vi "Subscribe_QMH.vi"() -> ()   [LabVIEW 2015]
uses:
  Program Files/National Instruments/LabVIEW 2015/ProjectTemplates/Source/Core/Queued Message Handler/support/Message Queue/Subscribe_Data.ctl
  <vilib>/daq.io/MQTT LabVIEW Client/Controls/QoS.ctl
  <vilib>/daq.io/MQTT LabVIEW Client/Controls/Connect_Flags.ctl
  <vilib>/daq.io/MQTT LabVIEW Client/Controls/DUP_Flag.ctl
  <vilib>/daq.io/MQTT LabVIEW Client/Controls/Retain_Flag.ctl
  <vilib>/daq.io/MQTT LabVIEW Client/Controls/Connection_Return_Codes.ctl
  Data_Save.ctl
  Program Files/National Instruments/LabVIEW 2015/ProjectTemplates/Source/Core/Queued Message Handler/support/Message Queue/Enqueue Message (Single).vi
  <vilib>/Utility/error.llb/Error Cluster From Error Code.vi
  <vilib>/ErrorRing/Error Ring.xnode
  Program Files/National Instruments/LabVIEW 2015/ProjectTemplates/Source/Core/Queued Message Handler/support/User Event - Stop/User Event - Stop.lvlib
  Program Files/National Instruments/LabVIEW 2015/ProjectTemplates/Source/Core/Queued Message Handler/support/Message Queue/Message Queue.lvlib
  <vilib>/daq.io/MQTT LabVIEW Client/MQTT_Functions.lvlib
panel:
  in  "append to file? (new file:F)":bool=TRUE
  out "Published Data":string[][](array[string])
  out "Samples Collected":i32
  in  "Sample Period(s)":dbl=1.0
  out "Connection Status":T1=enum."Connection refused: not authorized"
  out "Main Display":string
  in  "?":T2={"Subscriber ID"="GETmyRIO", "MQTT Broker"={"address (IP)"="52.37.169.179", "port"=1883}, "Subscription Info Array"=[{"Topic"="a/b", "QoS"=enum."At least once"}], "Connect Flags"={"user name"=FALSE, "password"=FALSE, "will retain"=FALSE, "will flag"=FALSE, "clean session"=TRUE, "reserved"=FALSE, "will QoS"=enum."At most once"}, "Connect Meta"={"QoS"=enum."At most once", "DUP"=FALSE, "Retain"=FALSE, "Keep Alive (sec)"=60}, "Exit"=refnum, "connection ID out"=refnum, "Main Display"=""}
  in  "Exit":bool
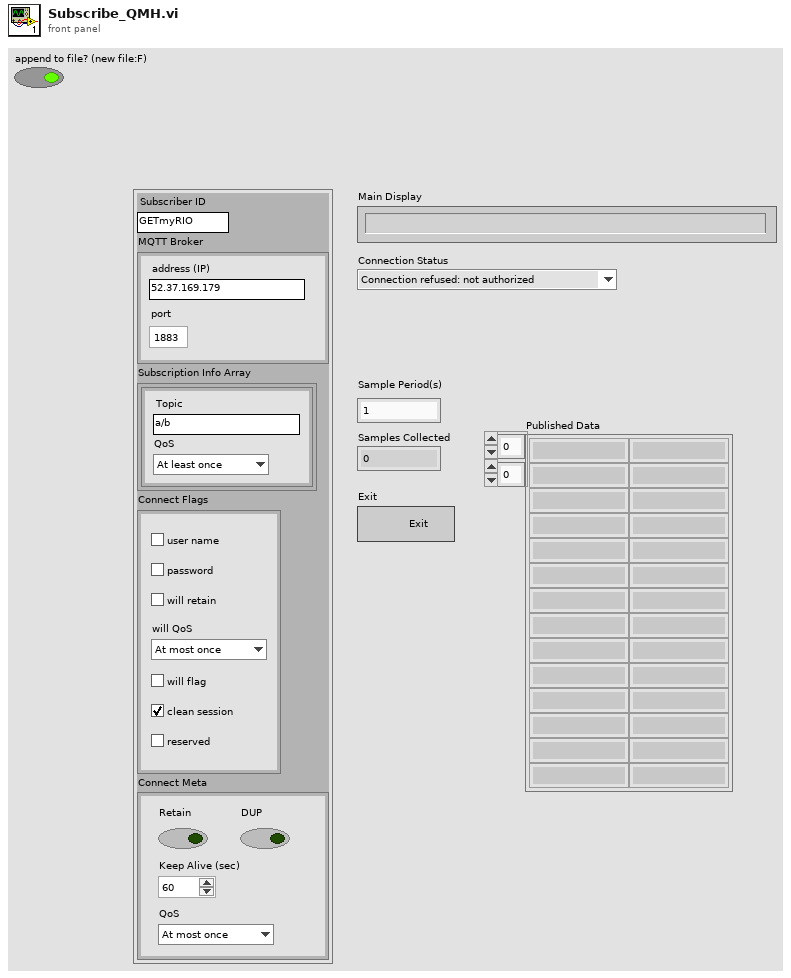
[diagram p1: front panel]
types:
  T1 = typedef "MQTT_Functions.lvlib/Connection_Return_Codes.ctl" = enum16{"Connection accepted", "Connection refused: unacceptable protocol version", "Connection refused: identifier rejected", "Connection refused: Server unavailable", "Connection refused: bad user name or password", "Connection refused: not authorized"}
  T2 = typedef "Subscribe_Data.ctl" = cluster{"Subscriber ID":string, "MQTT Broker":cluster{"address (IP)":string, "port":u16}, "Subscription Info Array":cluster{"Topic":string, "QoS":T3}[], "Connect Flags":T4, "Connect Meta":cluster{"QoS":T3, "DUP":T5, "Retain":T6, "Keep Alive (sec)":u16}, "Exit":refnum<vi>, "connection ID out":refnum<k5>, "Main Display":string}
  T3 = typedef "MQTT_Functions.lvlib/QoS.ctl" = enum8{"At most once", "At least once", "Exactly once", "Reserved"}
  T4 = typedef "MQTT_Functions.lvlib/Connect_Flags.ctl" = cluster{"user name":bool, "password":bool, "will retain":bool, "will flag":bool, "clean session":bool, "reserved":bool, "will QoS":T3}
  T5 = typedef "MQTT_Functions.lvlib/DUP_Flag.ctl" = bool
  T6 = typedef "MQTT_Functions.lvlib/Retain_Flag.ctl" = bool
  T7 = typedef "Data_Save.ctl" = cluster{"Data Columns":string, "Raw Data":string, "file path (dialog if empty)":path, "Append File":refnum<vi>}
  T8 = typedef "Queues.ctl" = cluster{"Suscribe":refnum<queue>, "Display/Save Data":refnum<queue>}
  T9 = cluster{"QoS":T3, "DUP":T5, "Retain":T6, "Keep Alive (sec)":u16}
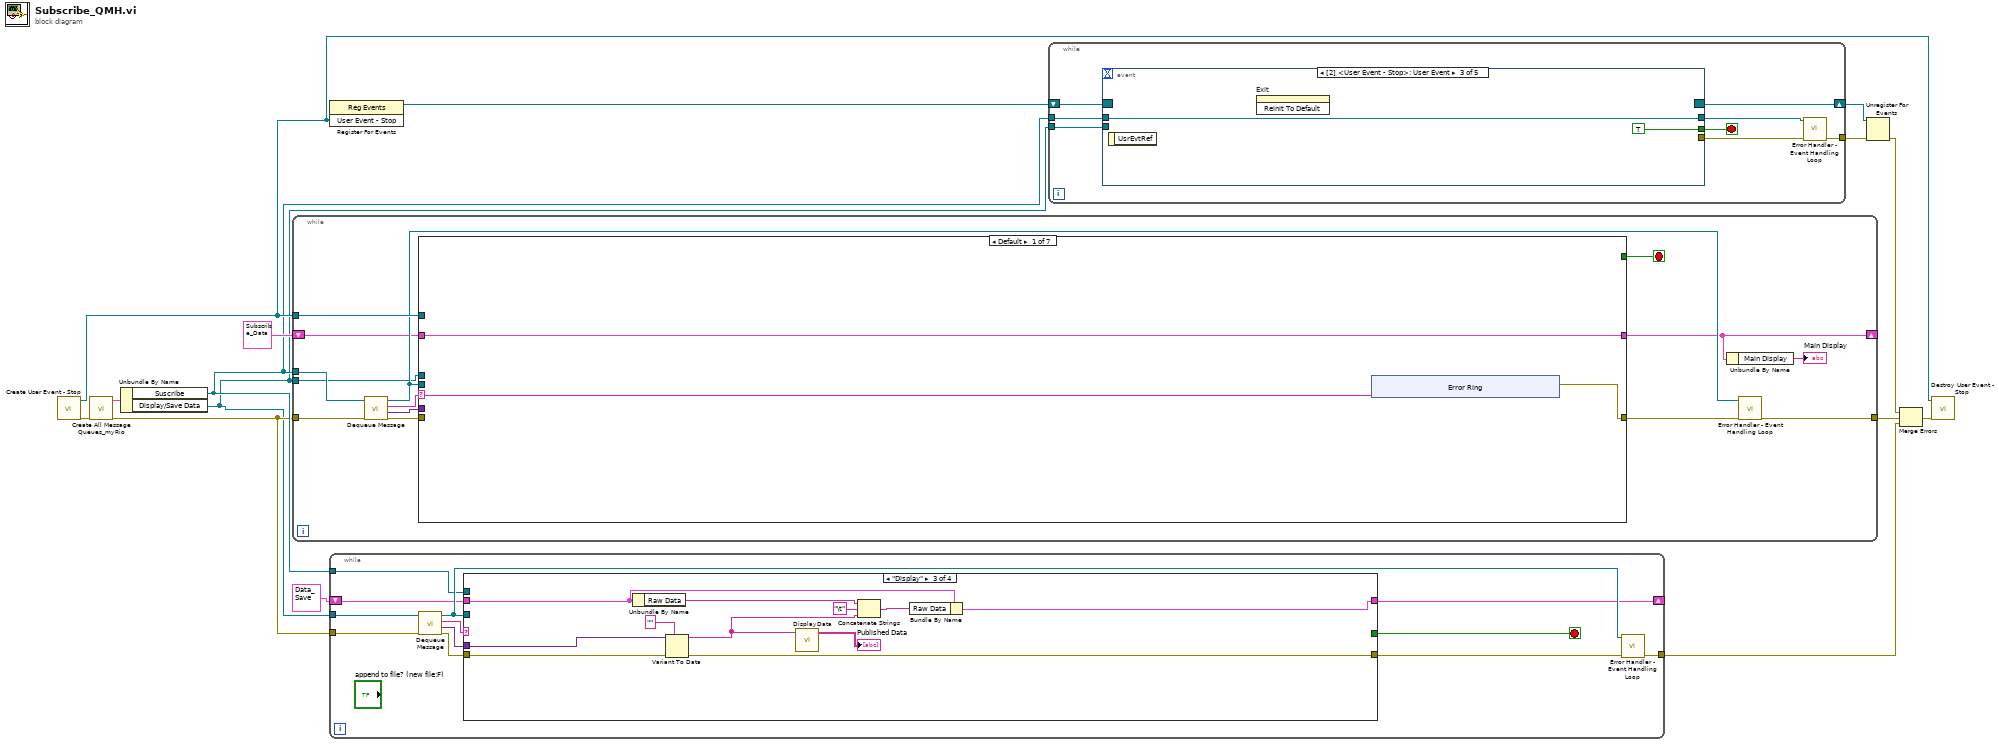
[diagram p0: block diagram]
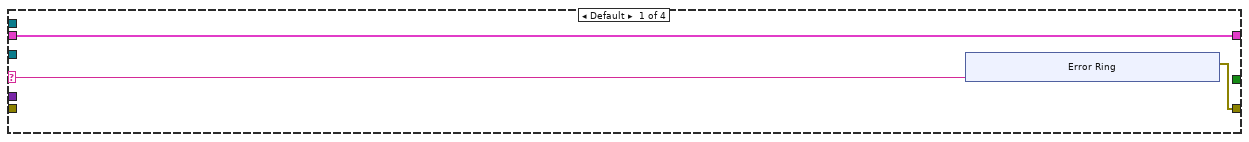
[diagram p2: hidden frame]
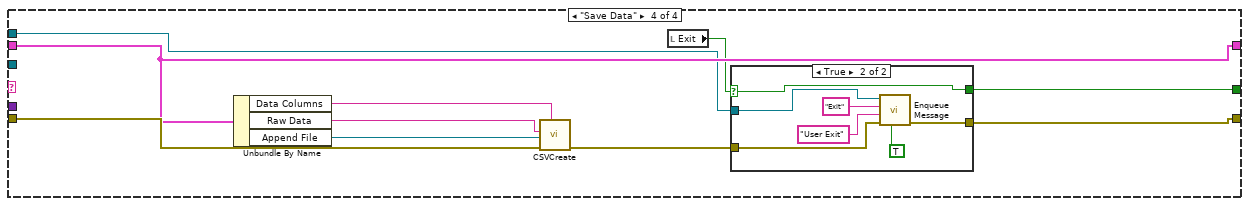
[diagram p4: hidden frame]
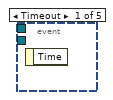
[diagram p6: hidden frame]
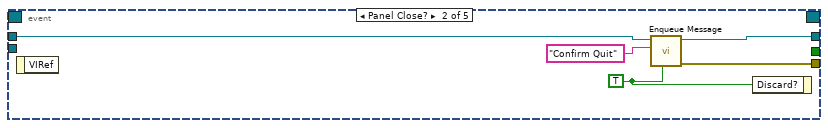
[diagram p7: hidden frame]
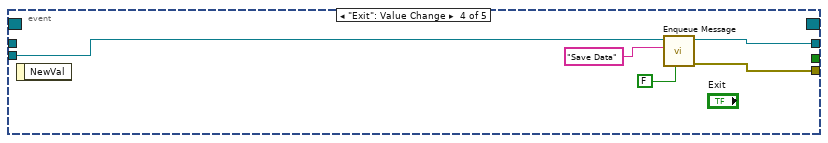
[diagram p8: hidden frame]
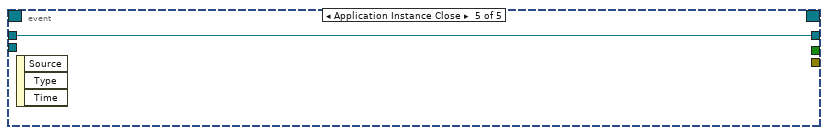
[diagram p9: hidden frame]
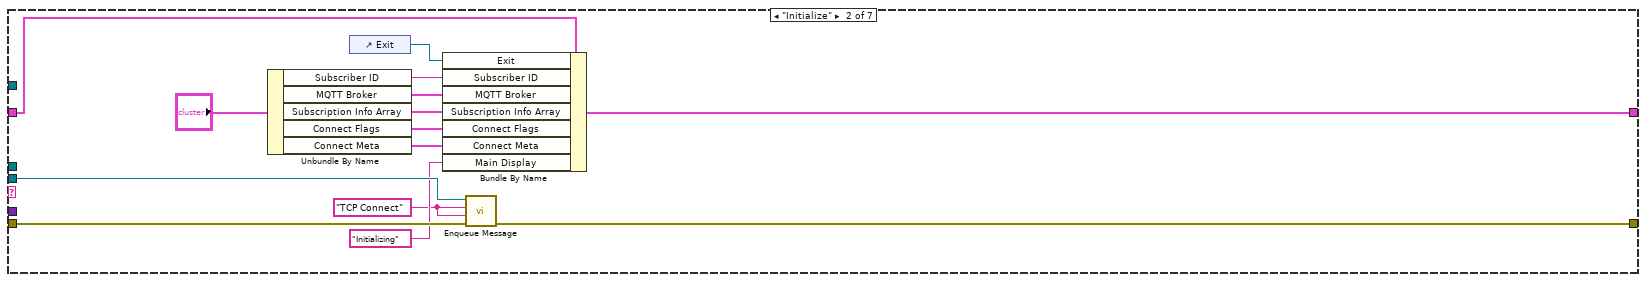
[diagram p10: hidden frame]
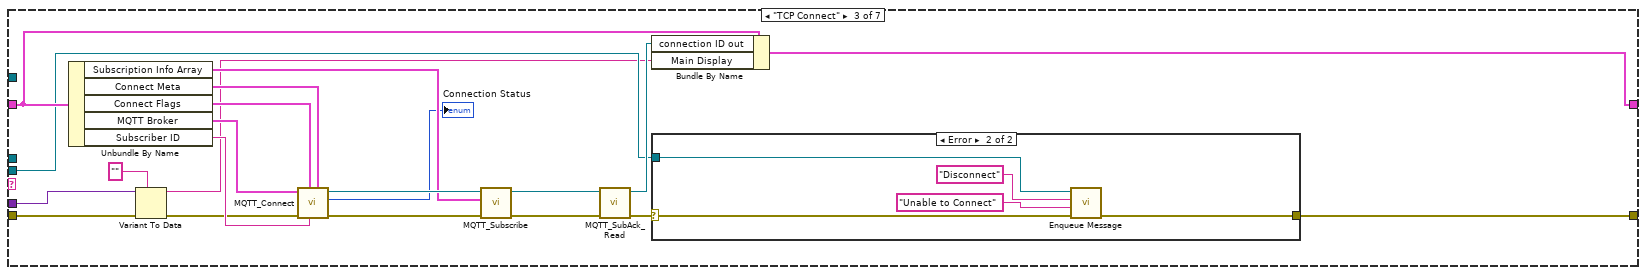
[diagram p11: hidden frame]
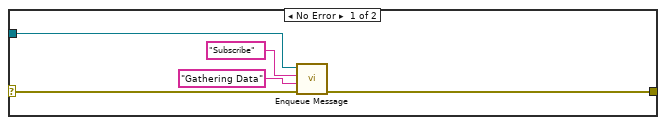
[diagram p12: hidden frame]
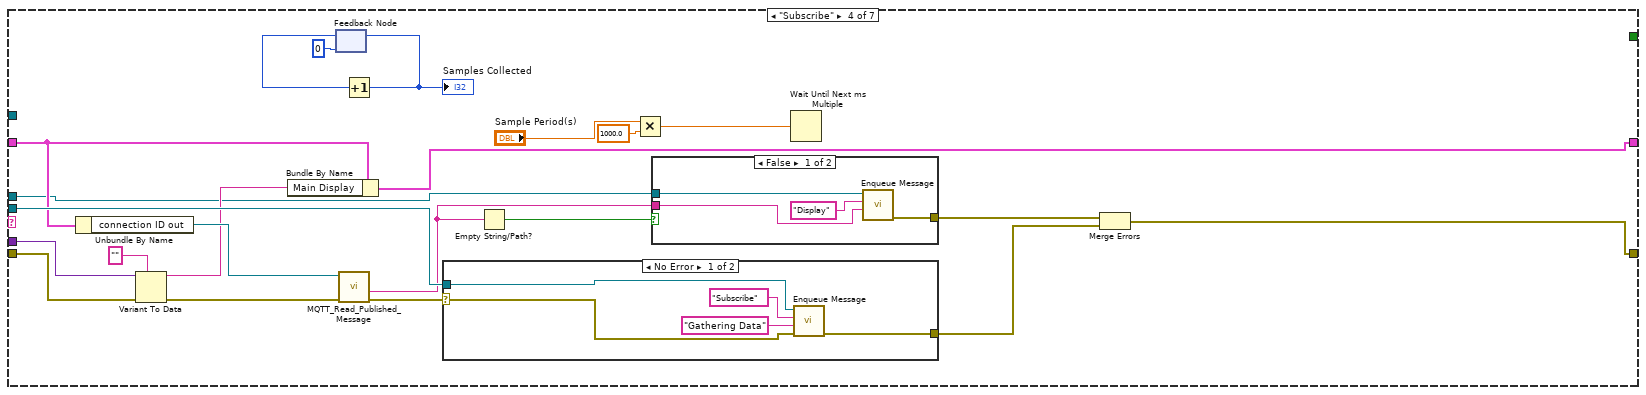
[diagram p13: hidden frame]
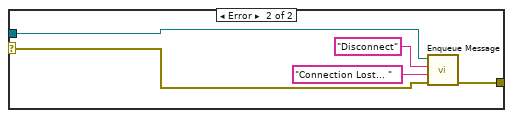
[diagram p14: hidden frame]
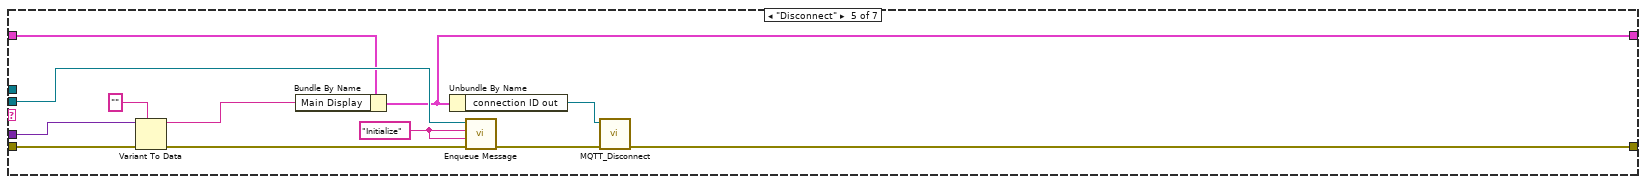
[diagram p16: hidden frame]
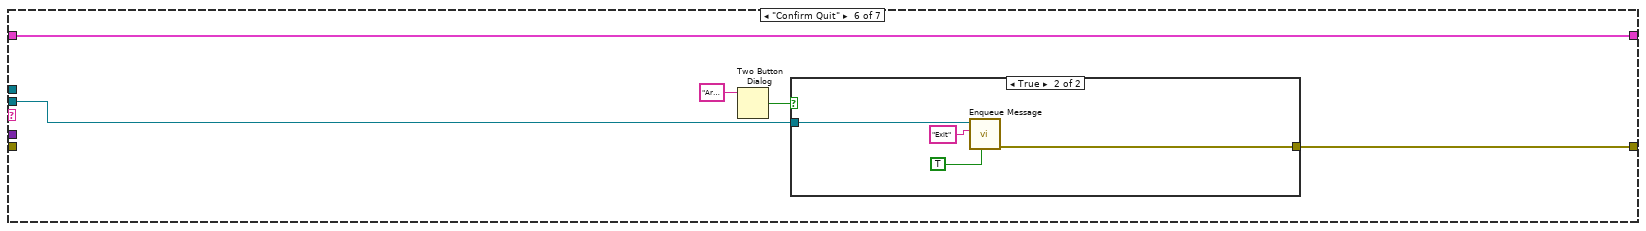
[diagram p17: hidden frame]
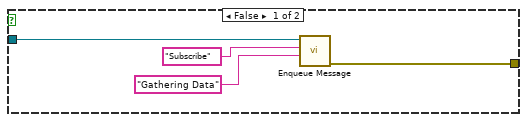
[diagram p18: hidden frame]
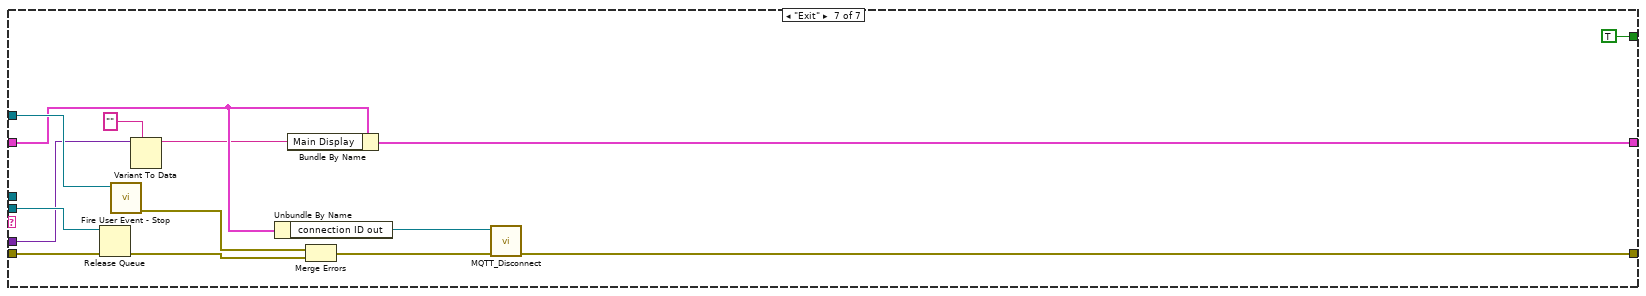
[diagram p19: hidden frame]
diagram:
  n1 = call "Create User Event - Stop.vi"() -> ("error out"=w15:errorcluster, "User Event - Stop"=w6:refnum<user-event>)  [unwired: 10 in]
  n2 = call "Create All Message Queues_myRio.vi"("error in (no error)"=w15) -> ("error out"=w4:errorcluster, "Queues"=w7:T8)  [unwired: 9 in]
  n3 = Unbundle By Name(w7) -> ("Suscribe"=w5:refnum<queue>, "Display/Save Data"=w1:refnum<queue>)
  n4 = while {
    tunnel: w4 -> [w29]
    tunnel: [w28] -> w9
    tunnel: w6 -> [w25]
    shift-right: [w18] -> _
    shift-left: T2 {"Subscriber ID"="GETmyRIO", "MQTT Broker"={"address (IP)"="52.37.169.179", "port"=1883}, "Subscription Info Array"=[{"Topic"="a/b", "QoS"=enum."At least once"}], "Connect Flags"={"user name"=FALSE, "password"=FALSE, "will retain"=FALSE, "will flag"=FALSE, "clean session"=TRUE, "reserved"=FALSE, "will QoS"=enum."At most once"}, "Connect Meta"={"QoS"=enum."At most once", "DUP"=FALSE, "Retain"=FALSE, "Keep Alive (sec)"=60}, "Exit"=refnum, "connection ID out"=refnum, "Main Display"=""} -> [w20]
    tunnel: w5 -> [w19]
    tunnel: w1 -> [w16]
    stop <- w22 stop-if-true
    n5 = call "Dequeue Message.vi"("error in (no error)"=w29, "Message Queue"=w19) -> ("error out"=w23:errorcluster, "Message Data"=w27:variant, "Message"=w26:string, "dup Message Queue"=w24:refnum<queue>)  [unwired: 6 in]
    n6 = case shown="Default" w26 {
      selector: w26 -> [w32 _ _ _ _ _ _]
      tunnel: w27 -> [_ _ w58 w92 w127 _ w150]
      tunnel: w25 -> [_ _ _ _ _ _ w159]
      tunnel: w24 -> [_ w44 w60 w101 w130 w137 w158]
      tunnel: w23 -> [_ w43 w57 w97 w125 _ w157]
      tunnel: [_ _ _ _ _ _ TRUE] -> w22
      tunnel: [w31 w42 w59 w99 w131 w136 w152] -> w21
      tunnel: w20 -> [w30 w52 w63 w94 w122 w133 w148]
      tunnel: [w30 w51 w62 w93 w121 w133 w147] -> w18
      tunnel: w16 -> [_ _ _ w87 _ _ _]
      frame Default {
        n7 = xnode "Error Ring"("parameter 0"=w32) -> ("error out"=w31:errorcluster)
      }
      frame "Initialize" {
        w40 = "TCP Connect" ("Message")
        n8 = Unbundle By Name("?") -> ("Subscriber ID"=w49:string, "MQTT Broker"=w48:cluster{"address (IP)":string, "port":u16}, "Subscription Info Array"=w47:cluster{"Topic":string, "QoS":T3}[], "Connect Flags"=w46:T4, "Connect Meta"=w45:T9)
        n9 = control-ref of="Exit"() -> (w53:refnum<vi>)
        n10 = Bundle By Name(cluster=w52, "Exit"=w53, "Subscriber ID"=w49, "MQTT Broker"=w48, "Subscription Info Array"=w47, "Connect Flags"=w46, "Connect Meta"=w45, "Main Display"="Initializing" ("Message")) -> (w51:T2)
        n11 = call-poly "Enqueue Message.vi"("error in (no error)"=w43, "Message Data"=w40, "Message"=w40, "Message Queue"=w44) -> ("error out"=w42:errorcluster)  [unwired: 6 in, 1 out]
      }
      frame "TCP Connect" {
        n12 = Unbundle By Name(w63) -> ("Subscription Info Array"=w66:cluster{"Topic":string, "QoS":T3}[], "Connect Meta"=w67:T9, "Connect Flags"=w68:T4, "MQTT Broker"=w69:cluster{"address (IP)":string, "port":u16}, "Subscriber ID"=w70:string)
        n13 = Variant To Data(error in=w57, type="", Variant=w58) -> (data=w55:string, error out=w54:errorcluster)
        n14 = call <vilib>:"MQTT_Connect.vi"("Connect Meta"=w67, "Client ID"=w70, "Connect Flags"=w68, "error in (no error)"=w54, "MQTT Broker"=w69) -> ("error out"=w72:errorcluster, "Connection Status"=→"Connection Status":T1, "connection ID out"=w71:refnum<k5>)  [unwired: 4 in]
        n15 = call <vilib>:"MQTT_Subscribe.vi"("error in (no error)"=w72, "Subscription Info Array"=w66, "connection ID"=w71) -> ("error out"=w74:errorcluster, "connection ID out"=w73:refnum<k5>)  [unwired: 7 in]
        n16 = call <vilib>:"MQTT_SubAck_Read.vi"("error in (no error)"=w74, "connection ID"=w73) -> ("error out"=w61:errorcluster, "connection ID out"=w64:refnum<k5>)  [unwired: 7 in, 1 out]
        n17 = Bundle By Name(cluster=w63, "connection ID out"=w64, "Main Display"=w55) -> (w62:T2)
        n18 = case shown="Error" w61 {
          selector: w61 -> [w77 w83]
          tunnel: w60 -> [w78 w84]
          tunnel: [w76 w82] -> w59
          frame No Error {
            n19 = call-poly "Enqueue Message.vi"("error in (no error)"=w77, "Message Data"="Gathering Data" ("Message"), "Message"="Subscribe", "Message Queue"=w78) -> ("error out"=w76:errorcluster)  [unwired: 6 in, 1 out]
          }
          frame Error {
            n20 = call-poly "Enqueue Message.vi"("error in (no error)"=w83, "Message Data"="Unable to Connect" ("Message"), "Message"="Disconnect", "Message Queue"=w84) -> ("error out"=w82:errorcluster)  [unwired: 6 in, 1 out]
          }
        }
      }
      frame "Subscribe" {
        n21 = Unbundle By Name(w94) -> ("connection ID out"=w102:refnum<k5>)
        n22 = Variant To Data(error in=w97, type="", Variant=w92) -> (data=w95:string, error out=w96:errorcluster)
        n23 = Bundle By Name(cluster=w94, "Main Display"=w95) -> (w93:T2)
        n24 = feedback #1(0) -> (w104:i32)
        n25 = call <vilib>:"MQTT_Read_Published_Message.vi"("error in (no error)"=w96, "connection ID"=w102) -> ("error out"=w85:errorcluster, "Message"=w88:string)  [unwired: 4 in, 4 out]
        n26 = Increment(x=w104) -> (x+1=w105:i32)
        "Samples Collected" <- w105
        n27 = feedback-in #1(w105) -> ()
        n28 = case shown="No Error" w85 {
          selector: w85 -> [w108 w113]
          tunnel: w101 -> [w111 w116]
          tunnel: [w109 w115] -> w100
          frame No Error {
            n29 = call-poly "Enqueue Message.vi"("error in (no error)"=w108, "Message Data"="Gathering Data" ("Message"), "Message"="Subscribe", "Message Queue"=w111) -> ("error out"=w109:errorcluster)  [unwired: 6 in, 1 out]
          }
          frame Error {
            n30 = call-poly "Enqueue Message.vi"("error in (no error)"=w113, "Message Data"="Connection Lost... " ("Message"), "Message"="Disconnect", "Message Queue"=w116) -> ("error out"=w115:errorcluster)  [unwired: 6 in, 1 out]
          }
        }
        n31 = Empty String/Path?(string/path=w88) -> (empty?=w103:bool)
        n32 = Multiply(x="Sample Period(s)", y=1000.0 ("milliseconds to wait")) -> (x*y=w89:dbl)
        n33 = case shown="False" w103 {
          tunnel: w88 -> [w118 _]
          tunnel: w87 -> [w120 _]
          tunnel: [w117 _] -> w86
          frame False {
            n34 = call-poly "Enqueue Message.vi"("Message Data"=w118, "Message"="Display", "Message Queue"=w120) -> ("error out"=w117:errorcluster)  [unwired: 7 in, 1 out]
          }
          frame True {
          }
        }
        n35 = Wait Until Next ms Multiple(millisecond multiple=w89) -> ()  [unwired: 1 out]
        n36 = Merge Errors(w86, w100) -> (w99:errorcluster)
      }
      frame "Disconnect" {
        w128 = "Initialize" ("Message")
        n37 = Variant To Data(error in=w125, type="", Variant=w127) -> (data=w123:string, error out=w124:errorcluster)
        n38 = Bundle By Name(cluster=w122, "Main Display"=w123) -> (w121:T2)
        n39 = Unbundle By Name(w121) -> ("connection ID out"=w132:refnum<k5>)
        n40 = call-poly "Enqueue Message.vi"("error in (no error)"=w124, "Message Data"=w128, "Message"=w128, "Message Queue"=w130) -> ("error out"=w129:errorcluster)  [unwired: 6 in, 1 out]
        n41 = call <vilib>:"MQTT_Disconnect.vi"("error in (no error)"=w129, "connection ID"=w132) -> ("error out"=w131:errorcluster)  [unwired: 9 in]
      }
      frame "Confirm Quit" {
        n42 = Two Button Dialog(message="Are you sure you want to quit?") -> (T button?=w134:bool)  [unwired: 2 in]
        n43 = case shown="True" w134 {
          tunnel: w137 -> [w141 w145]
          tunnel: [w139 w143] -> w136
          frame False {
            n44 = call-poly "Enqueue Message.vi"("Message Data"="Gathering Data" ("Message"), "Message"="Subscribe", "Message Queue"=w141) -> ("error out"=w139:errorcluster)  [unwired: 7 in, 1 out]
          }
          frame True {
            n45 = call-poly "Enqueue Message.vi"("Priority Message? (F)"=TRUE, "Message"="Exit", "Message Queue"=w145) -> ("error out"=w143:errorcluster)  [unwired: 7 in, 1 out]
          }
        }
      }
      frame "Exit" {
        n46 = Release Queue(queue=w158, error in (no error)=w157) -> (error out=w155:errorcluster)  [unwired: 1 in, 2 out]
        n47 = call "Fire User Event - Stop.vi"("User Event - Stop"=w159) -> ("error out"=w156:errorcluster)  [unwired: 10 in]
        n48 = Variant To Data(type="", Variant=w150) -> (data=w146:string)  [unwired: 1 in, 1 out]
        n49 = Unbundle By Name(w148) -> ("connection ID out"=w151:refnum<k5>)
        n50 = Bundle By Name(cluster=w148, "Main Display"=w146) -> (w147:T2)
        n51 = Merge Errors(w156, w155) -> (w153:errorcluster)
        n52 = call <vilib>:"MQTT_Disconnect.vi"("error in (no error)"=w153, "connection ID"=w151) -> ("error out"=w152:errorcluster)  [unwired: 9 in]
      }
    }
    n53 = Unbundle By Name(w18) -> ("Main Display"=→"Main Display":string)
    n54 = call "Error Handler - Event Handling Loop.vi"("error in (no error)"=w21, "Message Queue"=w24) -> ("dup error in"=w28:errorcluster)  [unwired: 8 in, 1 out]
  }
  n55 = register-events(w6) -> (reference out=w14:refnum<event-registration>)  [unwired: 2 in, 1 out]
  n56 = while {
    tunnel: w1 -> [w171]
    tunnel: w5 -> [w160]
    tunnel: w4 -> [w170]
    tunnel: [w165] -> w3
    shift-right: [w162] -> _
    shift-left: T7 {"Data Columns"="Timestamp,Wind Direction,Wind Speed,Air Temperature,Internal Temperature,Relative Humidity,Air Pressure,Rain Accumulation, Rain Duration, Rain Intensity,Hail Duration, Hail Intensity, Supply Voltage, Solar Irradiance", "Raw Data"="", "file path (dialog if empty)"=path "C:/Users/jas921/Desktop/Labview Test Data/test.csv", "Append File"=refnum} ("Display/Save Data") -> [w163]
    stop <- w161 stop-if-true
    n57 = call "Dequeue Message.vi"("error in (no error)"=w170, "Message Queue"=w171) -> ("error out"=w169:errorcluster, "Message Data"=w168:variant, "Message"=w167:string, "dup Message Queue"=w164:refnum<queue>)  [unwired: 6 in]
    n58 = case shown="\"Display\"" w167 {
      selector: w167 -> [w174 _ _ _]
      tunnel: w169 -> [_ w183 w192 w204]
      tunnel: w168 -> [_ _ w193 _]
      tunnel: w164 -> [_ _ _ _]
      tunnel: [w173 w183 w184 w197] -> w166
      tunnel: w163 -> [w172 w182 w186 w203]
      tunnel: [w172 w182 w188 w203] -> w162
      tunnel: [_ _ _ w199] -> w161
      tunnel: w160 -> [_ _ _ w198]
      frame Default {
        n59 = xnode "Error Ring"("parameter 0"=w174) -> ("error out"=w173:errorcluster)
      }
      frame "Wait" {
      }
      frame "Display" {
        n60 = Unbundle By Name(w186) -> ("Raw Data"=w185:string)
        n61 = Variant To Data(error in=w192, type="", Variant=w193) -> (data=w189:string, error out=w184:errorcluster)
        n62 = call "DisplayData.vi"("CSV Input"=w189) -> ("Published Data"=→"Published Data":string[][])  [unwired: 10 in]
        n63 = Concatenate Strings(w185, "\t", w189) -> (w187:string)
        n64 = Bundle By Name(cluster=w186, "Raw Data"=w187) -> (w188:T7)
      }
      frame "Save Data" {
        n65 = Unbundle By Name(w203) -> ("Data Columns"=w202:string, "Raw Data"=w201:string, "Append File"=w195:refnum<vi>)
        n66 = call "CSVCreate.vi"("Header"=w202, "error in"=w204, "Append File"=w195, "Data Input"=w201) -> ("error out"=w196:errorcluster)  [unwired: 6 in, 1 out]
        n67 = local read "Exit"() -> (w200:bool)
        n68 = case shown="True" w200 {
          selector: w200 -> [_ w212]
          tunnel: [_ w212] -> w199
          tunnel: w198 -> [_ w211]
          tunnel: [w205 w208] -> w197
          tunnel: w196 -> [w205 w207]
          frame False {
          }
          frame True {
            n69 = call-poly "Enqueue Message.vi"("Priority Message? (F)"=TRUE, "error in (no error)"=w207, "Message Data"="User Exit" ("Message"), "Message"="Exit", "Message Queue"=w211) -> ("error out"=w208:errorcluster)  [unwired: 5 in, 1 out]
          }
        }
      }
    }
    n70 = call "Error Handler - Event Handling Loop.vi"("error in (no error)"=w166, "Message Queue"=w164) -> ("dup error in"=w165:errorcluster)  [unwired: 8 in, 1 out]
  }
  n71 = while {
    tunnel: w5 -> [w220]
    tunnel: [w217] -> w12
    shift-right: [w215] -> w13
    shift-left: w14 -> [w216]
    tunnel: w1 -> [w213]
    stop <- w214 stop-if-true
    n72 = event shown="[2] <User Event - Stop>: User Event" {
      selector: w216 -> [_ _ _ _ _]
      dyn-events: [_ _ _ _ _] -> w215
      timeout: _ -> [_ _ _ _ _]
      tunnel: w220 -> [_ w224 w226 _ w233]
      tunnel: [_ w223 w226 w232 w233] -> w219
      tunnel: [_ w222 _ w229 _] -> w218
      tunnel: [_ _ TRUE _ _] -> w214
      tunnel: w213 -> [_ _ _ w228 _]
      event Timeout {
        n73 = event-data() -> ()  [unwired: 1 in, 1 out]
      }
      event Panel Close? {
        w221 = TRUE
        n74 = event-data() -> ()  [unwired: 1 in, 1 out]
        n75 = call-poly "Enqueue Message.vi"("Priority Message? (F)"=w221, "Message"="Confirm Quit", "Message Queue"=w224) -> ("error out"=w222:errorcluster, "dup Message Queue"=w223:refnum<queue>)  [unwired: 7 in]
        n76 = event-data("Discard?"=w221) -> ()  [unwired: 1 in, 1 out]
      }
      event User Event {
        n77 = event-data() -> ()  [unwired: 1 in, 1 out]
        n78 = invoke on="Exit" class="Bool (strict)" method="Reinit To Default"() -> ()  [unwired: 3 in, 3 out]
      }
      event "Exit": Value Change {
        n79 = event-data() -> ()  [unwired: 1 in, 1 out]
        n80 = call-poly "Enqueue Message.vi"("Priority Message? (F)"=FALSE, "Message"="Save Data", "Message Queue"=w228) -> ("error out"=w229:errorcluster, "dup Message Queue"=w232:refnum<queue>)  [unwired: 7 in]
      }
      event Application Instance Close {
        n81 = event-data() -> ()  [unwired: 1 in, 3 out]
      }
    }
    n82 = call "Error Handler - Event Handling Loop.vi"("error in (no error)"=w218, "Message Queue"=w219) -> ("dup error in"=w217:errorcluster)  [unwired: 8 in, 1 out]
  }
  n83 = Unregister For Events(event registration refnum=w13, error in=w12) -> (error out=w11:errorcluster)
  n84 = Merge Errors(w11, w9, w3) -> (w10:errorcluster)
  n85 = call "Destroy User Event - Stop.vi"("error in (no error)"=w10, "User Event - Stop"=w6) -> ()  [unwired: 9 in, 1 out]
